vi "Close File.vi"(8 "error in (no error)":errorcluster, 10 "File Refnum":variant, 11 "TDMS File in":refnum<class "TDMS File.lvclass">) -> (0 "error out":errorcluster, 3 "TDMS File out":refnum<class "TDMS File.lvclass">)   [LabVIEW 2021, in "TDMS File.lvclass"]
doc: "This vi helps to close TDMS file."
uses:
  TDMS File.lvclass
  File Abstract Class/File Abstract.lvclass
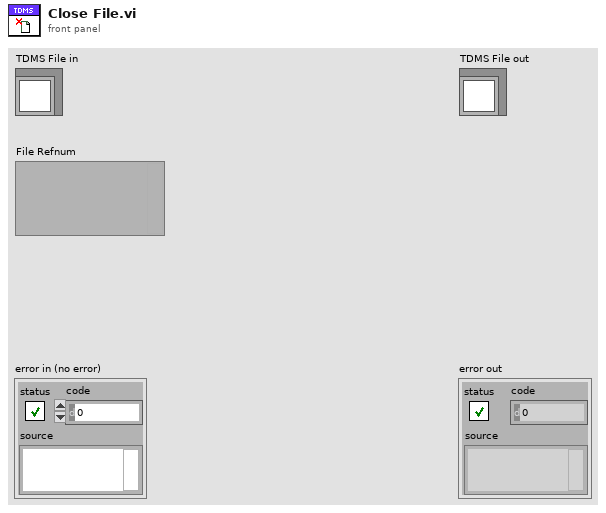
[diagram p1: front panel]
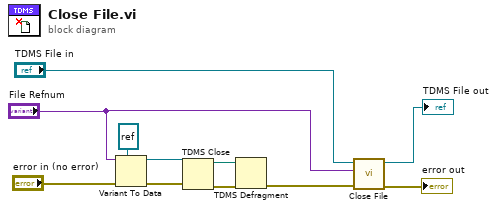
[diagram p0: block diagram]
diagram:
  n1 = Variant To Data(error in="error in (no error)", type=refnum<k34> refnum ("tdms Refnum"), Variant="File Refnum") -> (data=w8:refnum<k34>, error out=w7:errorcluster)
  n2 = TDMS Close(8:w7, 11:w8) -> (0:w3:errorcluster, 3:w2:path)
  n3 = TDMS Defragment(4:w3, 7:w2) -> (0:w1:errorcluster)
  n4 = call-parent "Close File.vi"("error in (no error)"=w1, "File Refnum"="File Refnum", "File Manager in"="TDMS File in") -> ("error out"=→"error out":errorcluster, "File Manager out"=→"TDMS File out":refnum<class "TDMS File.lvclass">)  [unwired: 7 in]
